vi "1553B_Msg.vi"(7 "Timeout(默认:5ms)":i32=5, 8 "error in":errorcluster, 9 "主备份选择":enum8{"主份", "备份"}(ring), 10 "unsigned byte array":u8[](array[numeric]), 11 "VISA资源名称":refnum<visa-resource-name>) -> (0 "error out 2":errorcluster, 1 "timeout":bool, 3 "VISAout":refnum<visa-resource-name>)   [LabVIEW 2012]
uses:
  com/TONGXUN/write32.vi
  com/TONGXUN/write8.vi
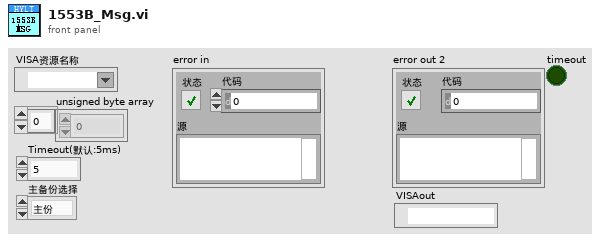
[diagram p1: front panel]
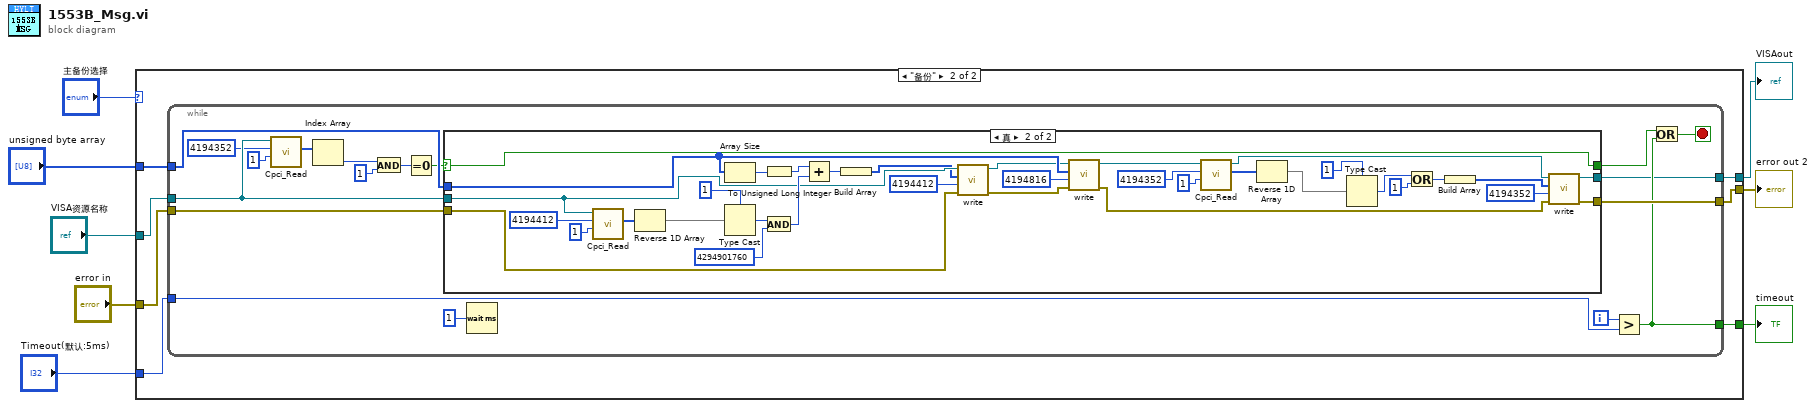
[diagram p0: block diagram]
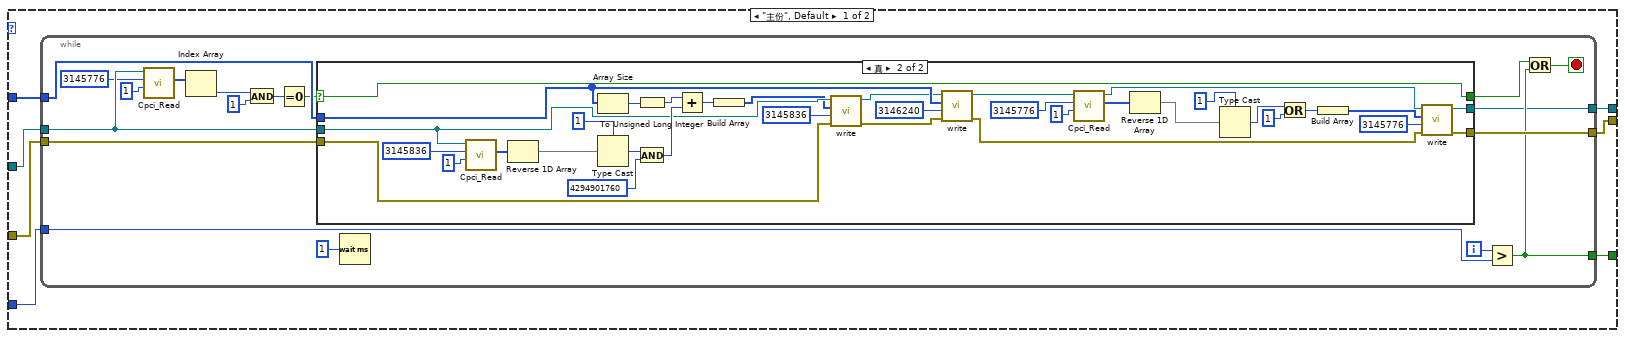
[diagram p2: hidden frame]
diagram:
  n1 = case shown="\"备份\"" "主备份选择" {
    tunnel: "VISA资源名称" -> [w15 w78]
    tunnel: "unsigned byte array" -> [w14 w77]
    tunnel: "error in" -> [w13 w76]
    tunnel: [w12 w75] -> w5
    tunnel: [w11 w74] -> w4
    tunnel: [w10 w73] -> w3
    tunnel: "Timeout(默认:5ms)" -> [w9 w72]
    frame "主份", Default {
      n2 = while {
        tunnel: w15 -> [w30]
        tunnel: w14 -> [w33]
        tunnel: w13 -> [w32]
        tunnel: [w31] -> w12
        tunnel: [w18] -> w11
        tunnel: [w17] -> w10
        tunnel: w9 -> [w16]
        i -> [w21]
        stop <- w20 stop-if-true
        n3 = call "Cpci_Read.vi"("u32_len"=1, "基地址"=u32 3145776, "VISA资源名称"=w30) -> ("U8"=w27:u8[])  [unwired: 6 in, 2 out]
        n4 = Index Array(array=w27) -> (element=w26:u8)  [unwired: 1 in]
        n5 = And(x=w26, y=u8 1) -> (x .and. y?=w24:u8)
        n6 = Equal To 0?(x=w24) -> (x = 0?=w23:bool)
        n7 = case shown="真" w23 {
          selector: w23 -> [w36 w63]
          tunnel: w30 -> [w34 w51]
          tunnel: w33 -> [_ w70]
          tunnel: w32 -> [w35 w67]
          tunnel: [w35 w64] -> w31
          tunnel: [w36 w63] -> w19
          tunnel: [w34 w61] -> w17
          frame False {
          }
          frame True {
            n8 = call "Cpci_Read.vi"("u32_len"=1, "基地址"=u32 3145836 ("偏移量(0)"), "VISA资源名称"=w51) -> ("U8"=w55:u8[])  [unwired: 6 in, 2 out]
            n9 = Reverse 1D Array(array=w55) -> (reversed array=w56:u8[])
            n10 = Array Size(array=w70) -> (size(s)=w49:i32)
            n11 = Type Cast(type=u32 1 ("u32_len"), x=w56) -> (*(type *) &x=w58:u32)
            n12 = To Unsigned Long Integer(number=w49) -> (unsigned 32bit integer=w53:u32)
            n13 = And(x=w58, y=u32 4294901760) -> (x .and. y?=w54:u32)
            n14 = Add(x=w53, y=w54) -> (x+y=w52:u32)
            n15 = Build Array(w52) -> (w48:u32[])
            n16 = call-poly "write.vi"("error out"=w67, "起始地址"=u32 3145836 ("偏移量(0)"), "U32"=w48, "VISA资源名称输入"=w51) -> ("error out 2"=w66:errorcluster, "VISA资源名称输出"=w62:refnum<visa-resource-name>)  [unwired: 6 in]
            n17 = call-poly "write.vi"("error out"=w66, "起始地址"=u32 3146240 ("偏移量(0)"), "数组"=w70, "VISA资源名称输入"=w62) -> ("error out 2"=w65:errorcluster, "VISA资源名称 输出"=w38:refnum<visa-resource-name>)  [unwired: 6 in]
            n18 = call "Cpci_Read.vi"("u32_len"=1, "基地址"=u32 3145776 ("偏移量(0)"), "VISA资源名称"=w38) -> ("U8"=w43:u8[], "VISA资源名称输出"=w37:refnum<visa-resource-name>)  [unwired: 6 in, 1 out]
            n19 = Reverse 1D Array(array=w43) -> (reversed array=w41:u8[])
            n20 = Type Cast(type=u32 1 ("u32_len"), x=w41) -> (*(type *) &x=w45:u32)
            n21 = Or(x=w45, y=u32 1) -> (x .or. y?=w40:u32)
            n22 = Build Array(w40) -> (w39:u32[])
            n23 = call-poly "write.vi"("error out"=w65, "起始地址"=u32 3145776 ("偏移量(0)"), "U32"=w39, "VISA资源名称输入"=w37) -> ("error out 2"=w64:errorcluster, "VISA资源名称输出"=w61:refnum<visa-resource-name>)  [unwired: 6 in]
          }
        }
        n24 = Wait (ms)(milliseconds to wait=u32 1 ("等待时间（毫秒）")) -> ()  [unwired: 1 out]
        n25 = Greater?(x=w21, y=w16) -> (0:w18:bool)
        n26 = Or(x=w19, y=w18) -> (x .or. y?=w20:bool)
      }
    }
    frame "备份" {
      n27 = while {
        tunnel: w78 -> [w93]
        tunnel: w77 -> [w96]
        tunnel: w76 -> [w95]
        tunnel: [w94] -> w75
        tunnel: [w81] -> w74
        tunnel: [w80] -> w73
        tunnel: w72 -> [w79]
        i -> [w84]
        stop <- w83 stop-if-true
        n28 = call "Cpci_Read.vi"("u32_len"=1, "基地址"=u32 4194352, "VISA资源名称"=w93) -> ("U8"=w90:u8[])  [unwired: 6 in, 2 out]
        n29 = Index Array(array=w90) -> (element=w89:u8)  [unwired: 1 in]
        n30 = And(x=w89, y=u8 1) -> (x .and. y?=w87:u8)
        n31 = Equal To 0?(x=w87) -> (x = 0?=w86:bool)
        n32 = case shown="真" w86 {
          selector: w86 -> [w99 w126]
          tunnel: w93 -> [w97 w114]
          tunnel: w96 -> [_ w133]
          tunnel: w95 -> [w98 w130]
          tunnel: [w98 w127] -> w94
          tunnel: [w99 w126] -> w82
          tunnel: [w97 w124] -> w80
          frame False {
          }
          frame True {
            n33 = call "Cpci_Read.vi"("u32_len"=1, "基地址"=u32 4194412 ("偏移量(0)"), "VISA资源名称"=w114) -> ("U8"=w118:u8[])  [unwired: 6 in, 2 out]
            n34 = Reverse 1D Array(array=w118) -> (reversed array=w119:u8[])
            n35 = Array Size(array=w133) -> (size(s)=w112:i32)
            n36 = Type Cast(type=u32 1 ("u32_len"), x=w119) -> (*(type *) &x=w121:u32)
            n37 = To Unsigned Long Integer(number=w112) -> (unsigned 32bit integer=w116:u32)
            n38 = And(x=w121, y=u32 4294901760) -> (x .and. y?=w117:u32)
            n39 = Add(x=w116, y=w117) -> (x+y=w115:u32)
            n40 = Build Array(w115) -> (w111:u32[])
            n41 = call-poly "write.vi"("error out"=w130, "起始地址"=u32 4194412 ("偏移量(0)"), "U32"=w111, "VISA资源名称输入"=w114) -> ("error out 2"=w129:errorcluster, "VISA资源名称输出"=w125:refnum<visa-resource-name>)  [unwired: 6 in]
            n42 = call-poly "write.vi"("error out"=w129, "起始地址"=u32 4194816 ("偏移量(0)"), "数组"=w133, "VISA资源名称输入"=w125) -> ("error out 2"=w128:errorcluster, "VISA资源名称 输出"=w101:refnum<visa-resource-name>)  [unwired: 6 in]
            n43 = call "Cpci_Read.vi"("u32_len"=1, "基地址"=u32 4194352 ("偏移量(0)"), "VISA资源名称"=w101) -> ("U8"=w106:u8[], "VISA资源名称输出"=w100:refnum<visa-resource-name>)  [unwired: 6 in, 1 out]
            n44 = Reverse 1D Array(array=w106) -> (reversed array=w104:u8[])
            n45 = Type Cast(type=u32 1 ("u32_len"), x=w104) -> (*(type *) &x=w108:u32)
            n46 = Or(x=w108, y=u32 1) -> (x .or. y?=w103:u32)
            n47 = Build Array(w103) -> (w102:u32[])
            n48 = call-poly "write.vi"("error out"=w128, "起始地址"=u32 4194352 ("偏移量(0)"), "U32"=w102, "VISA资源名称输入"=w100) -> ("error out 2"=w127:errorcluster, "VISA资源名称输出"=w124:refnum<visa-resource-name>)  [unwired: 6 in]
          }
        }
        n49 = Wait (ms)(milliseconds to wait=u32 1 ("等待时间（毫秒）")) -> ()  [unwired: 1 out]
        n50 = Greater?(x=w84, y=w79) -> (0:w81:bool)
        n51 = Or(x=w82, y=w81) -> (x .or. y?=w83:bool)
      }
    }
  }
  "error out 2" <- w5
  "timeout" <- w4
  "VISAout" <- w3
